vi "Data(Analysis).vi"(0 "当前状态":string, 1 "读取缓冲区":string, 2 "最近三次读取缓存":string[](array[string])) -> (7 "当前状态":string, 8 "更新曲线":bool)   [LabVIEW 2020, in "人体健康监测系统.lvclass"]
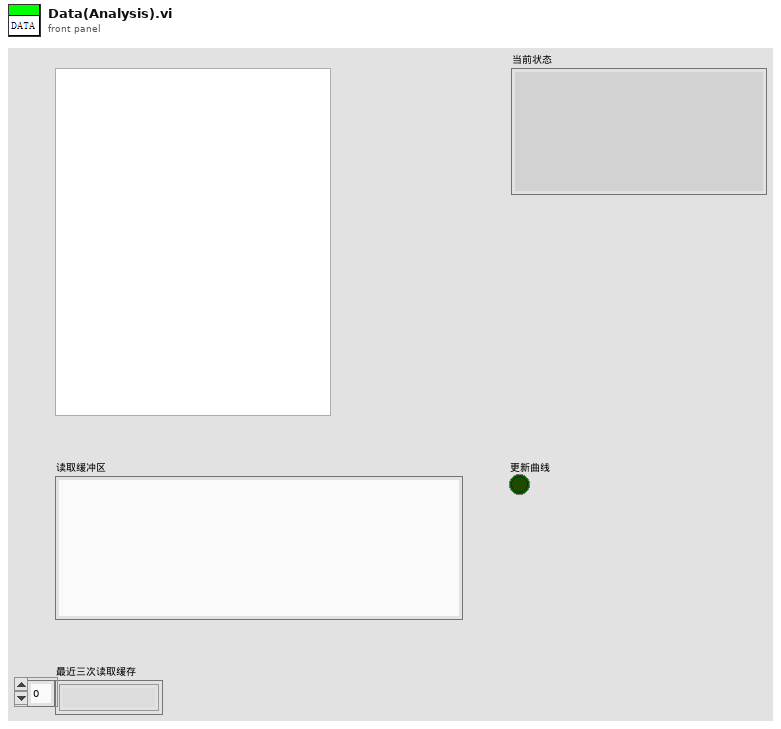
[diagram p1: front panel]
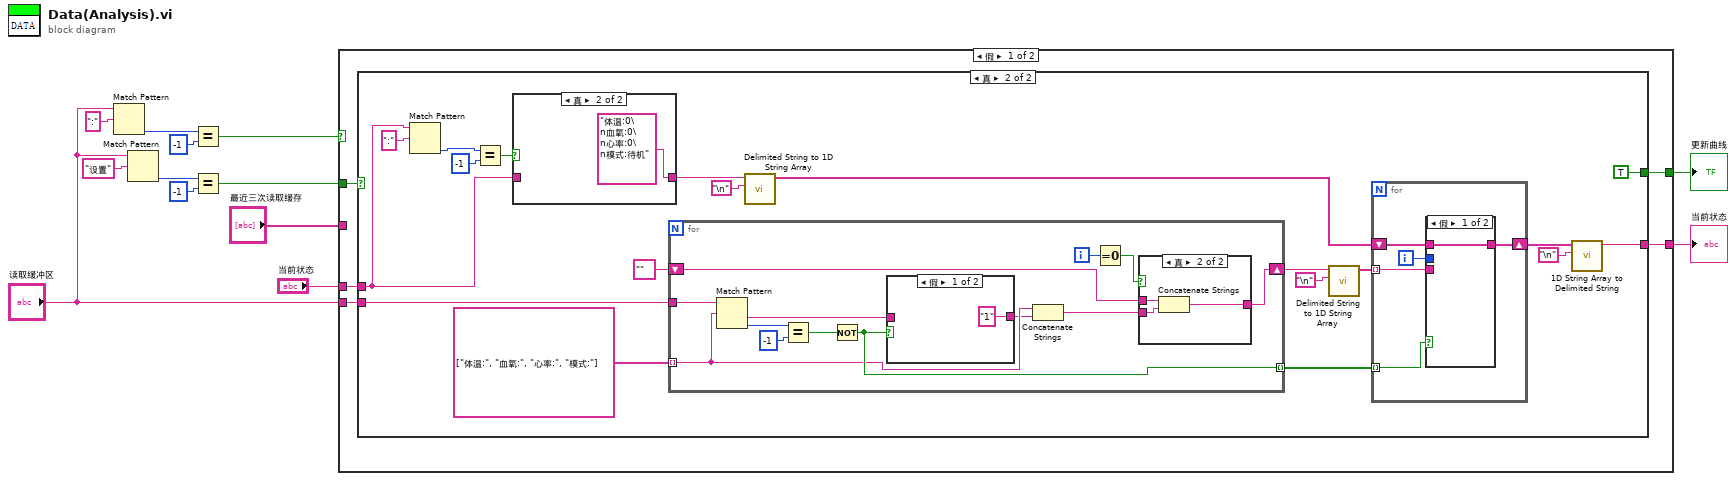
[diagram p0: block diagram]
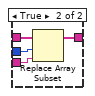
[diagram p3: hidden frame]
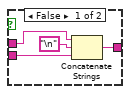
[diagram p5: hidden frame]
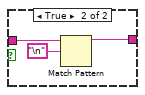
[diagram p6: hidden frame]
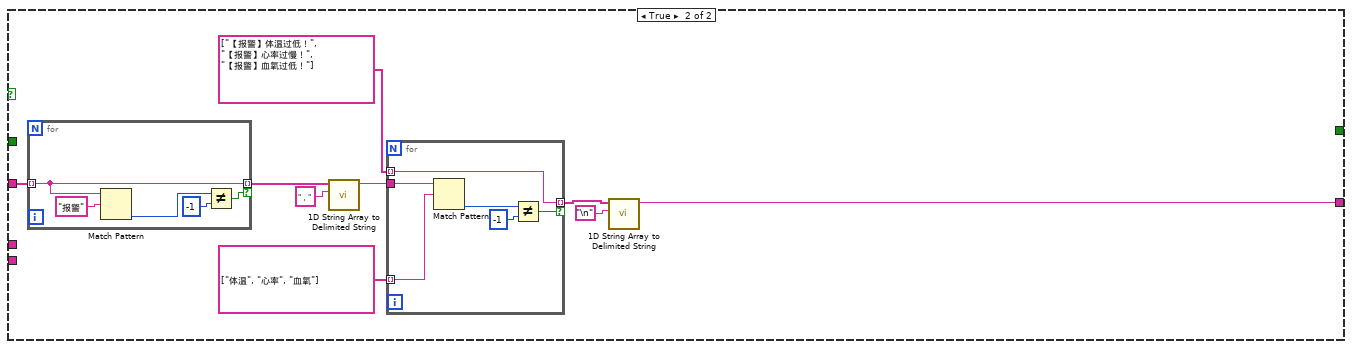
[diagram p7: hidden frame]
diagram:
  n1 = Match Pattern(string="读取缓冲区", regular expression=":" ("正则表达式")) -> (offset past match=w12:i32)  [unwired: 1 in, 3 out]
  n2 = Match Pattern(string="读取缓冲区", regular expression="设置" ("正则表达式")) -> (offset past match=w5:i32)  [unwired: 1 in, 3 out]
  n3 = Equal?(x=w12, y=-1) -> (x = y?=w4:bool)
  n4 = Equal?(x=w5, y=-1) -> (x = y?=w3:bool)
  n5 = case shown="假" w4 {
    tunnel: "当前状态" -> [w17 _]
    tunnel: "读取缓冲区" -> [w18 _]
    tunnel: [w16 w75] -> w9
    tunnel: w3 -> [w15 _]
    tunnel: [w14 _] -> w2
    tunnel: "最近三次读取缓存" -> [_ w83]
    frame False {
      n6 = case shown="真" w15 {
        tunnel: w18 -> [w19 w37]
        tunnel: w17 -> [_ w32]
        tunnel: [w19 w21] -> w16
        tunnel: [_ TRUE ("更新曲线")] -> w14
        frame False {
        }
        frame True {
          n7 = Match Pattern(string=w32, regular expression=":" ("正则表达式")) -> (offset past match=w34:i32)  [unwired: 1 in, 3 out]
          n8 = Equal?(x=w34, y=-1) -> (x = y?=w33:bool)
          n9 = case shown="真" w33 {
            tunnel: [w49 "体温:0\n血氧:0\n心率:0\n模式:待机"] -> w31
            tunnel: w32 -> [w49 _]
            frame False {
            }
            frame True {
            }
          }
          n10 = for {
            tunnel: string[] ["体温:", "血氧:", "心率:", "模式:"] -> [w53] mode=indexing
            tunnel: w37 -> [w63]
            shift-right: [w55] -> w27
            shift-left: "" ("读取缓冲区") -> [w58]
            tunnel: [w54] -> w25 mode=indexing
            i -> [w57]
            n11 = Match Pattern(string=w63, regular expression=w53) -> (after substring=w59:string, offset past match=w62:i32)  [unwired: 1 in, 2 out]
            n12 = Equal?(x=w62, y=-1) -> (x = y?=w60:bool)
            n13 = Not(x=w60) -> (.not. x?=w54:bool)
            n14 = case shown="假" w54 {
              tunnel: w59 -> [_ w74]
              tunnel: ["1" ("读取缓冲区") w72] -> w52
              frame False {
              }
              frame True {
                n15 = Match Pattern(string=w74, regular expression="\n") -> (before substring=w72:string)  [unwired: 1 in, 3 out]
              }
            }
            n16 = Concatenate Strings(w53, w52) -> (w51:string)
            n17 = Equal To 0?(x=w57) -> (x = 0?=w56:bool)
            n18 = case shown="真" w56 {
              tunnel: w58 -> [w67 w70]
              tunnel: w51 -> [w65 w69]
              tunnel: [w64 w68] -> w55
              frame False {
                n19 = Concatenate Strings(w67, "\n", w65) -> (w64:string)
              }
              frame True {
                n20 = Concatenate Strings(w70, w69) -> (w68:string)
              }
            }
          }
          n21 = call <vilib>:"Delimited String to 1D String Array.vi"("delimiter"="\n", "delimited string"=w31) -> ("string array"=w26:string[])  [unwired: 9 in]
          n22 = call <vilib>:"Delimited String to 1D String Array.vi"("delimiter"="\n", "delimited string"=w27) -> ("string array"=w24:string[])  [unwired: 9 in]
          n23 = for {
            shift-right: [w42] -> w23
            shift-left: w26 -> [w43]
            tunnel: w25 -> [w40] mode=indexing
            tunnel: w24 -> [w39] mode=indexing
            i -> [w41]
            n24 = case shown="假" w40 {
              tunnel: w43 -> [w44 w48]
              tunnel: [w44 w47] -> w42
              tunnel: w41 -> [_ w46]
              tunnel: w39 -> [_ w45]
              frame False {
              }
              frame True {
                n25 = Replace Array Subset(array=w48, new element=w45, index=w46) -> (w47:string[])
              }
            }
          }
          n26 = call <vilib>:"1D String Array to Delimited String.vi"("delimiter"="\n", "string array"=w23) -> ("delimited string"=w21:string)  [unwired: 9 in]
        }
      }
    }
    frame True {
      n27 = for {
        tunnel: w83 -> [w91] mode=indexing
        tunnel: [w91] -> w82 mode=indexing if=w90
        n28 = Match Pattern(string=w91, regular expression="报警" ("正则表达式")) -> (offset past match=w93:i32)  [unwired: 1 in, 3 out]
        n29 = Not Equal?(x=w93, y=-1) -> (x != y?=w90:bool)
      }
      n30 = call <vilib>:"1D String Array to Delimited String.vi"("delimiter"="，", "string array"=w82) -> ("delimited string"=w80:string)  [unwired: 9 in]
      n31 = for {
        tunnel: w80 -> [w89]
        tunnel: string[] ["体温", "心率", "血氧"] -> [w88] mode=indexing
        tunnel: string[] ["【报警】体温过低！", "【报警】心率过慢！", "【报警】血氧过低！"] -> [w85] mode=indexing
        tunnel: [w85] -> w77 mode=indexing if=w84
        n32 = Match Pattern(string=w89, regular expression=w88) -> (offset past match=w86:i32)  [unwired: 1 in, 3 out]
        n33 = Not Equal?(x=w86, y=-1) -> (x != y?=w84:bool)
      }
      n34 = call <vilib>:"1D String Array to Delimited String.vi"("delimiter"="\n", "string array"=w77) -> ("delimited string"=w75:string)  [unwired: 9 in]
    }
  }
  "当前状态" <- w9
  "更新曲线" <- w2
